vi "detect connected chassis.vi"(8 "error in":errorcluster, 11 "SysCfg Session in":refnum<k21>) -> (0 "error out":errorcluster, 2 "Chassis":T2 {"Remote Chassis"."Product ID" format="%.0x"; "Local Chassis"."Product ID" format="%.0x"}, 3 "SysCfg Session out":refnum<k21>)   [LabVIEW 2016, in "SMI.lvlib" / "Controller.lvclass"]
uses:
  Controller.lvclass
  Chassis/Controls/ChassisInformation.ctl
  <vilib>/nisyscfg/Close (System).vi
  <vilib>/nisyscfg/Close (Filter).vi
  <vilib>/nisyscfg/Close (Resources).vi
  <resource>/objmgr/niflexriosae.rc
  <resource>/objmgr/nicriosae.rc
  <vilib>/nisyscfg/nisyscfg.lvlib
  <resource>/objmgr/nisysapi.rc
  Chassis/Chassis.lvclass
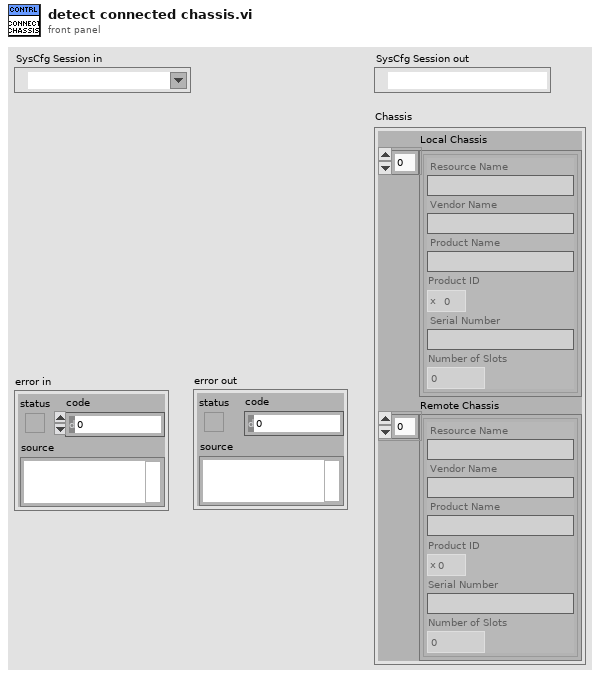
[diagram p1: front panel]
types:
  T1 = typedef "SMI.lvlib/Chassis.lvclass/ChassisInformation.ctl" = cluster{"Resource Name":string, "Vendor Name":string, "Product Name":string, "Product ID":u16, "Serial Number":string, "Number of Slots":i32}
  T2 = cluster{"Local Chassis":T1[], "Remote Chassis":T1[]}
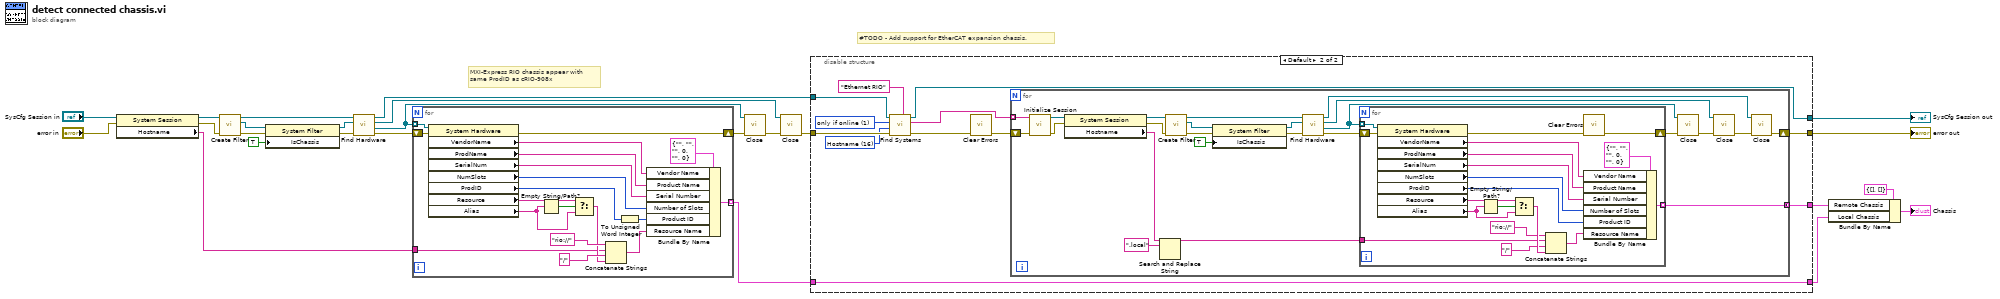
[diagram p0: block diagram]
diagram:
  # "#TODO - Add support for EtherCAT expansion chassis."
  # "MXI-Express RIO chassis appear with\nsame ProdID as cRIO-908x"
  n1 = property class="System Session"(reference="SysCfg Session in", error in="error in") -> (reference out=w7:refnum<k21>, error out=w6:errorcluster, "Hostname"=w5:string)
  n2 = call <vilib>:"Create Filter.vi"("error in (no error)"=w6, "Session in"=w7) -> ("error out"=w4:errorcluster, "Filter out"=w3:refnum<k20>, "Session out"=w17:refnum<k21>)  [unwired: 7 in]
  n3 = property class="System Filter"(reference=w3, error in=w4, "IsChassis"=TRUE ("Is Chassis")) -> (reference out=w16:refnum<k20>, error out=w15:errorcluster)
  n4 = call <vilib>:"Find Hardware.vi"("error in (no error)"=w15, "Filter in"=w16, "Session in"=w17) -> ("error out"=w14:errorcluster, "Resources out"=w11:refnum<k20>[], "Filter out"=w10:refnum<k20>, "Session out"=w8:refnum<k21>)  [unwired: 5 in]
  n5 = for {
    tunnel: w11 -> [w44] mode=indexing
    shift-right: [w41] -> w12
    shift-left: w14 -> [w43]
    tunnel: [w42] -> w1 mode=indexing
    tunnel: w5 -> [w29]
    n6 = property class="System Hardware"(reference=w44, error in=w43) -> (error out=w41:errorcluster, "VendorName"=w40:string, "ProdName"=w39:string, "SerialNum"=w38:string, "NumSlots"=w37:i32, "ProdID"=w26:u32, "Resource"=w31:string, "Alias"=w32:string)  [unwired: 1 out]
    n7 = Empty String/Path?(string/path=w32) -> (empty?=w33:bool)
    n8 = Select(t=w31, s=w33, f=w32) -> (s? t:f=w30:string)
    n9 = Concatenate Strings("rio://" ("string"), w29, "/" ("string"), w30) -> (w36:string)
    n10 = To Unsigned Word Integer(number=w26) -> (unsigned 16bit integer=w27:u16)
    n11 = Bundle By Name(cluster=T1 {"Resource Name"="", "Vendor Name"="", "Product Name"="", "Product ID"=0, "Serial Number"="", "Number of Slots"=0} ("Chassis Information"), "Vendor Name"=w40, "Product Name"=w39, "Serial Number"=w38, "Number of Slots"=w37, "Product ID"=w27, "Resource Name"=w36) -> (w42:T1)
  }
  n12 = call-poly <vilib>:"Close.vi"("error in (no error)"=w12, "Resources in"=w11) -> ("error out"=w13:errorcluster)  [unwired: 9 in]
  n13 = call-poly <vilib>:"Close.vi"("error in (no error)"=w13, "Filter in"=w10) -> ("error out"=w9:errorcluster)  [unwired: 9 in]
  n14 = disable-structure shown="Default" {
    disable-tunnel: w1 -> [w45 w48]
    disable-tunnel: w9 -> [w47 w59]
    disable-tunnel: w8 -> [w46 w58]
    disable-tunnel: [w47 w56] -> w25
    disable-tunnel: [_ w49] -> w20
    disable-tunnel: [w46 w50] -> w22
    disable-tunnel: [w45 w48] -> w19
    frame condition #0 {
      # "Possible CAR: PharLap and VxWorks targets cannot detect Ethernet RIO chassis using Find Systems.vi."
    }
    frame condition #1 (active) {
      w54 = u32 1 items=["none"=0, "only if online"=1, "all"=3] ("Include Cached Results (all)")
      w55 = u32 16 items=["Hostname"=16, "Hostname (IP)"=18, "Hostname (MAC)"=19, "IP"=32, "IP (Hostname)"=33, "IP (MAC)"=35, "MAC"=48, "MAC (Hostname)"=49, "MAC (IP)"=50] ("Output (Hostname and IP)")
      n15 = call <vilib>:"Find Systems.vi"("Device Class"="Ethernet RIO", "error in (no error)"=w59, "Output (Hostname and IP)"=w55, "Include Cached Results (all)"=w54, "Session in (localhost)"=w58) -> ("error out"=w51:errorcluster, "Detected Systems"=w57:string[], "Session out"=w50:refnum<k21>)  [unwired: 4 in]
      n16 = call <vilib>:"Clear Errors.vi"("error in (no error)"=w51) -> ("error out"=w52:errorcluster)  [unwired: 5 in, 1 out]
      n17 = for {
        shift-right: [w72] -> w56
        shift-left: w52 -> [w83]
        tunnel: [w74] -> w49 mode=concatenating
        tunnel: w57 -> [w70] mode=indexing
        n18 = call <vilib>:"Initialize Session.vi"("error in (no error)"=w83, "Target (localhost)"=w70) -> ("error out"=w67:errorcluster, "Session out"=w69:refnum<k21>)  [unwired: 8 in]
        n19 = property class="System Session"(reference=w69, error in=w67) -> (reference out=w68:refnum<k21>, error out=w66:errorcluster, "Hostname"=w65:string)
        n20 = Search and Replace String(input string=w65, search string=".local") -> (result string=w64:string)  [unwired: 6 in, 3 out]
        n21 = call <vilib>:"Create Filter.vi"("error in (no error)"=w66, "Session in"=w68) -> ("error out"=w60:errorcluster, "Filter out"=w61:refnum<k20>, "Session out"=w75:refnum<k21>)  [unwired: 7 in]
        n22 = property class="System Filter"(reference=w61, error in=w60, "IsChassis"=TRUE ("Is Chassis")) -> (reference out=w76:refnum<k20>, error out=w77:errorcluster)
        n23 = call <vilib>:"Find Hardware.vi"("error in (no error)"=w77, "Filter in"=w76, "Session in"=w75) -> ("error out"=w78:errorcluster, "Resources out"=w81:refnum<k20>[], "Filter out"=w82:refnum<k20>, "Session out"=w73:refnum<k21>)  [unwired: 5 in]
        n24 = for {
          tunnel: w81 -> [w102] mode=indexing
          shift-right: [w93] -> w80
          shift-left: w78 -> [w101]
          tunnel: [w100] -> w74 mode=indexing
          tunnel: w64 -> [w85]
          n25 = property class="System Hardware"(reference=w102, error in=w101) -> (error out=w94:errorcluster, "VendorName"=w99:string, "ProdName"=w98:string, "SerialNum"=w97:string, "NumSlots"=w96:i32, "ProdID"=w95:u32, "Resource"=w87:string, "Alias"=w86:string)  [unwired: 1 out]
          n26 = Empty String/Path?(string/path=w86) -> (empty?=w91:bool)
          n27 = Select(t=w87, s=w91, f=w86) -> (s? t:f=w92:string)
          n28 = Concatenate Strings("rio://" ("string"), w85, "/" ("string"), w92) -> (w88:string)
          n29 = Bundle By Name(cluster=T1 {"Resource Name"="", "Vendor Name"="", "Product Name"="", "Product ID"=0, "Serial Number"="", "Number of Slots"=0} ("Chassis Information"), "Vendor Name"=w99, "Product Name"=w98, "Serial Number"=w97, "Number of Slots"=w96, "Product ID"=w95, "Resource Name"=w88) -> (w100:T1)
          n30 = call <vilib>:"Clear Errors.vi"("error in (no error)"=w94) -> ("error out"=w93:errorcluster)  [unwired: 5 in, 1 out]
        }
        n31 = call-poly <vilib>:"Close.vi"("error in (no error)"=w80, "Resources in"=w81) -> ("error out"=w79:errorcluster)  [unwired: 9 in]
        n32 = call-poly <vilib>:"Close.vi"("error in (no error)"=w79, "Filter in"=w82) -> ("error out"=w71:errorcluster)  [unwired: 9 in]
        n33 = call-poly <vilib>:"Close.vi"("error in (no error)"=w71, "Session in"=w73) -> ("error out"=w72:errorcluster)  [unwired: 9 in]
      }
    }
  }
  "error out" <- w25
  "SysCfg Session out" <- w22
  n34 = Bundle By Name(cluster=T2 {"Local Chassis"=[], "Remote Chassis"=[]} ("Chassis"), "Remote Chassis"=w20, "Local Chassis"=w19) -> (→"Chassis":T2)
